vi "csvdecode.vi"(11 "file path (dialog if empty)":path) -> (0 "Time":dbl[](array[numeric]), 1 "Quantity":dbl[](array[numeric]), 2 "Message":string[](array[string]), 3 "Name":string[](array[string]))   [LabVIEW 2018]
uses:
  <vilib>/Utility/file.llb/Read Delimited Spreadsheet (string).vi
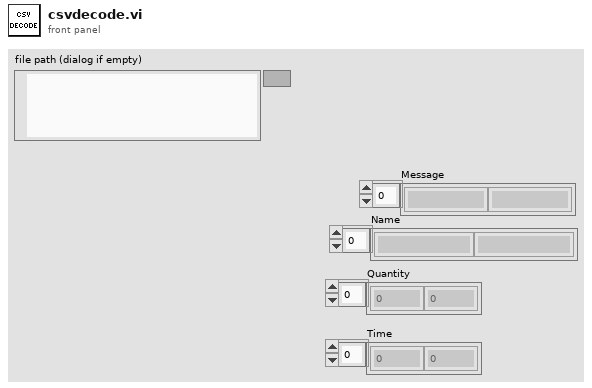
[diagram p1: front panel]
types:
  T1 = cluster{"Name":string, "time":string, "message":string, "quantity":dbl}
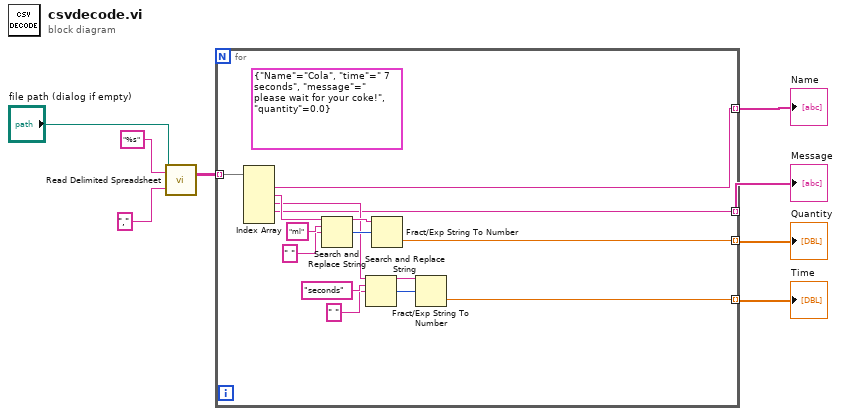
[diagram p0: block diagram]
diagram:
  n1 = call-poly <vilib>:"Read Delimited Spreadsheet.vi"("file path (dialog if empty)"="file path (dialog if empty)", "format (%s)"="%s", "delimiter (\\t)"="," ("delimiter (\\t)")) -> ("all rows"=w6:string[][])  [unwired: 7 in, 5 out]
  n2 = for {
    tunnel: w6 -> [w23] mode=indexing
    tunnel: [w12] -> w5 mode=indexing
    tunnel: [w11] -> w2 mode=indexing
    tunnel: [w10] -> w3 mode=indexing
    tunnel: [w9] -> w4 mode=indexing
    (unwired) T1 {"Name"="Cola", "time"=" 7 seconds", "message"=" please wait for your coke!", "quantity"=0.0} ("Cluster")
    n3 = Index Array(array=w23) -> (element #1=w9:string, element #2=w22:string, element #3=w13:string, element #4=w12:string)  [unwired: 5 in, 1 out]
    n4 = Search and Replace String(input string=w22, search string="ml", replace string=" " ("replace string (\"\")")) -> (result string=w18:string, number of replacements=w19:i32)  [unwired: 5 in, 2 out]
    n5 = Search and Replace String(input string=w13, search string="seconds", replace string=" " ("replace string (\"\")")) -> (result string=w17:string, number of replacements=w16:i32)  [unwired: 5 in, 2 out]
    n6 = Fract/Exp String To Number(string=w18, offset=w19) -> (number=w10:dbl)  [unwired: 2 in, 1 out]
    n7 = Fract/Exp String To Number(string=w17, offset=w16) -> (number=w11:dbl)  [unwired: 2 in, 1 out]
  }
  "Message" <- w5
  "Name" <- w4
  "Quantity" <- w3
  "Time" <- w2
